vi "Set Factory Pattern.vi"(11 "Funcion":string) -> (3 "Clase":refnum<class "Generador.lvclass">)   [LabVIEW 2020, in "FGen.lvlib"]
uses:
  FGen.lvlib
  Generador/Generador.lvclass
  GeneradorAmplificado/GeneradorAmplificado.lvclass
  C:/Users/HP/Documents/7mo/Instrumentacion/Examen_2doParcial/IV2Parcial-develop/Libraries/FGen/Generador/Generador.lvclass
panel:
  out "Clases":string[](array[string])
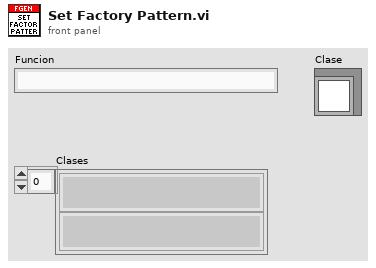
[diagram p1: front panel]
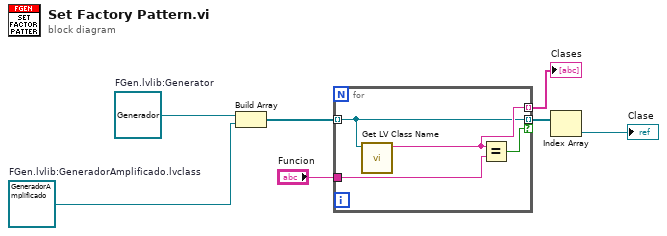
[diagram p0: block diagram]
diagram:
  w4 = refnum<class "GeneradorAmplificado.lvclass"> refnum  # FGen.lvlib:GeneradorAmplificado.lvclass
  w3 = refnum<class "Generador.lvclass"> refnum  # FGen.lvlib:Generator
  n1 = Build Array "Build Array"(w3, w4) -> (w6:refnum<class "Generador.lvclass">[])
  n2 = for {
    tunnel: w6 -> [w9] mode=indexing
    tunnel: [w10] -> w2 mode=indexing
    tunnel: "Funcion" -> [w11]
    tunnel: [w9] -> w7 mode=indexing if=w8
    n3 = call <vilib>:"Get LV Class Name.vi"("object"=w9) -> ("class name"=w10:string)  [unwired: 9 in, 1 out]
    n4 = Equal?(x=w10, y=w11) -> (x = y?=w8:bool)
  }
  "Clases" <- w2
  n5 = Index Array "Index Array"(array=w7) -> (element=→"Clase":refnum<class "Generador.lvclass">)  [unwired: 1 in]
